vi "Timing.vi"(1 "start time (s)":timestamp) -> (0 "last reading (s)":timestamp)   [LabVIEW 2016]
uses:
  Instrument_Setup.vi
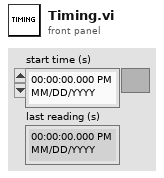
[diagram p1: front panel]
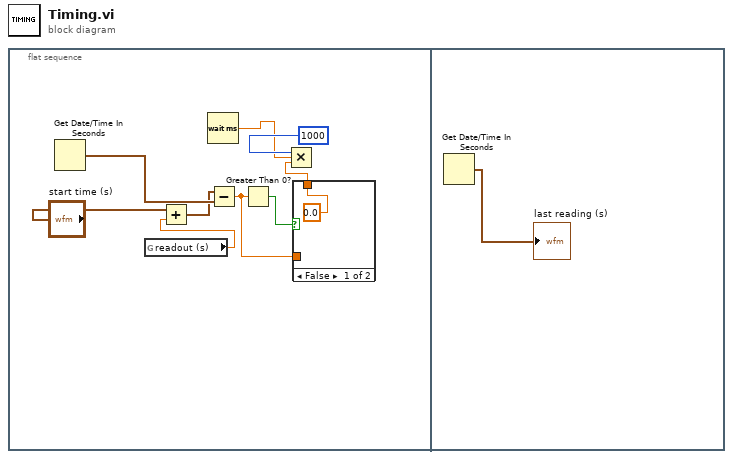
[diagram p0: block diagram]
diagram:
  n1 = flat-sequence {
    frame #0 {
      n2 = Get Date/Time In Seconds() -> (seconds since 1Jan1904=w6:timestamp)
      n3 = global read "Instrument_Setup.vi" "readout (s)"() -> (w7:dbl)
      n4 = Add(x="start time (s)", y=w7) -> (x+y=w5:timestamp)
      n5 = Subtract(x=w5, y=w6) -> (x-y=w3:dbl)
      n6 = Greater Than 0?(x=w3) -> (x > 0?=w4:bool)
      n7 = case shown="False" w4 {
        tunnel: w3 -> [_ w11]
        tunnel: [0.0 w11] -> w2
        frame False {
        }
        frame True {
        }
      }
      n8 = Multiply(x=1000, y=w2) -> (x*y=w8:dbl)
      n9 = Wait (ms)(milliseconds to wait=w8) -> ()  [unwired: 1 out]
    }
    frame #1 {
      n10 = Get Date/Time In Seconds() -> (seconds since 1Jan1904=→"last reading (s)":timestamp)
    }
  }
